vi "Main.vi"() -> ()   [LabVIEW 2018]
uses:
  MainFrame/TypeDefs/DisplayCluster.ctl
  MainFrame/TypeDefs/CiscoStats.ctl
  MainFrame/TypeDefs/Command_Enum.ctl
  ModulesDS/TypeDefs/PR_Parameters.ctl
  MainFrame/TypeDefs/FGV_Enum.ctl
  MainFrame/TypeDefs/InternalDataCluster.ctl
  Modules/Private Controls/Report Data Cluster.ctl
  Modules/Private Controls/Data Raw.ctl
  ModulesDS/GetNeglectedSRs.vi
  ModulesDS/GetOpenSRs.vi
  MainFrame/MainFrameLib.lvlib
  Modules/Data Operations.lvlib
  ModulesDS/SRReportParser.lvlib
  ModulesDS/SRNotesParser/SRNotesParser.lvlib
panel:
  in  "Tab Control":T1(tab)=enum."Debug\\Configure"
  in  "Stop":bool
  in  "Refresh CISCO Agents":bool
  out "AEs List":i32(listbox)
  in  "UpdateReports":bool
  in  "New AEs":string(combo)
  in  "Configure AE Name Mapping":bool
  in  "Cancel Request":bool
  in  "Clear Folder":bool
  out "Report Available":bool
  in  "Load existing report":bool
  in  "Request Oracle Report":bool
  out "Available weeks":string
  out "Request ID":string="45252303"
  out "Cisco Stats":T2[](array[typedef])=[{"Agent Name"="Akos Hegedus", "Number"="4091404", "State"="Logged Off", "Time in state"="-", "Ready ?"=FALSE}, {"Agent Name"="Alin Balanescu", "Number"="4091454", "State"="Ready", "Time in state"="01:06:36", "Ready ?"=TRUE}, {"Agent Name"="Ambrus Gregor", "Number"="4091431", "State"="Logged Off", "Time in state"="-", "Ready ?"=FALSE}, {"Agent Name"="Andrzej Filipek", "Number"="4091443", "State"="Ready", "Time in state"="00:16:58", "Ready ?"=TRUE}, {"Agent Name"="Denis Stavila", "Number"="4283512", "State"="Logged Off", "Time in state"="-", "Ready ?"=FALSE}, {"Agent Name"="Filip Pribyl", "Number"="4025617", "State"="Ready", "Time in state"="00:00:22", "Ready ?"=TRUE}, {"Agent Name"="Kamil Gierczyk", "Number"="4091512", "State"="Ready", "Time in state"="00:00:18", "Ready ?"=TRUE}, {"Agent Name"="Lukas Wiesner", "Number"="4023029", "State"="Logged Off", "Time in state"="-", "Ready ?"=FALSE}, {"Agent Name"="Michal Jadrny", "Number"="4025611", "State"="Logged Off", "Time in state"="-", "Ready ?"=FALSE}, {"Agent Name"="Patrik Karandusovsky", "Number"="4025621", "State"="Not Ready", "Time in state"="18:54:40", "Ready ?"=FALSE}, {"Agent Name"="Tamas Virag", "Number"="4091437", "State"="Ready", "Time in state"="00:07:00", "Ready ?"=TRUE}, {"Agent Name"="Tomasz Kachnic", "Number"="4091455", "State"="Logged Off", "Time in state"="-", "Ready ?"=FALSE}, {"Agent Name"="Tomasz Kowalczyk", "Number"="4091463", "State"="Ready", "Time in state"="00:17:46", "Ready ?"=TRUE}]
  out "Update Required?":bool
  out "State":T3=enum."Shutdown"
  in  "Available Reports":i32(listbox)=-1
  in  "Year":i16=1904 min=1904 max=1904 step=1
  in  "Week":i16 min=1 max=52 step=1
  in  "Excel Report":bool
  out "Open SRs":u32(colorbox)=16711680
  out "Solved in more then 5 workdays":u32(colorbox)=16753962
  out "In work":u32(colorbox)=9567230
  out "Solved within 5 workdays":u32(colorbox)=6618880
  out "New SRs":u32(colorbox)=16860
  out "SR Data":string[][](array[string])
  out "Data Display":T4[](array[typedef]) {"Open SRs" scale=0.0..40.0; "Solved in more then 5 Workdays" scale=0.0..40.0; "In Work SRs" scale=0.0..40.0; "Solved Within 5 workdays" scale=0.0..40.0; "New SRs" scale=0.0..40.0}
  in  "Team Stats":bool
  in  "SR Summary":string(tree)
  in  "Filter by AE Name":string(combo)="Alin Balanescu"
  in  "SaveNeglectedToFile":bool
  in  "Neglected SRs":string(tree)="3161536"
  in  "Open SRs":string(tree)="3191694"
  in  "AEs Overview":T5(array[cluster]) {"SRs # (Graphical)" max=350 step=1 scale=0.0..100.0}
  out "Documents Linked":string[][](table)
  out "Documents marked as solution":string[][](table)
  out "SR Notes":string[](array[string])
  in  "KCS Links":bool
  in  "SR View":string(tree)
  out "AE Statistics":string[][](table)
  in  "Get Performance Data":bool
  in  "Configuration":T6
  in  "EmailAddress:":string="tamas.virag@ni.com" caption="@ni.com"
  out "error out":errorcluster
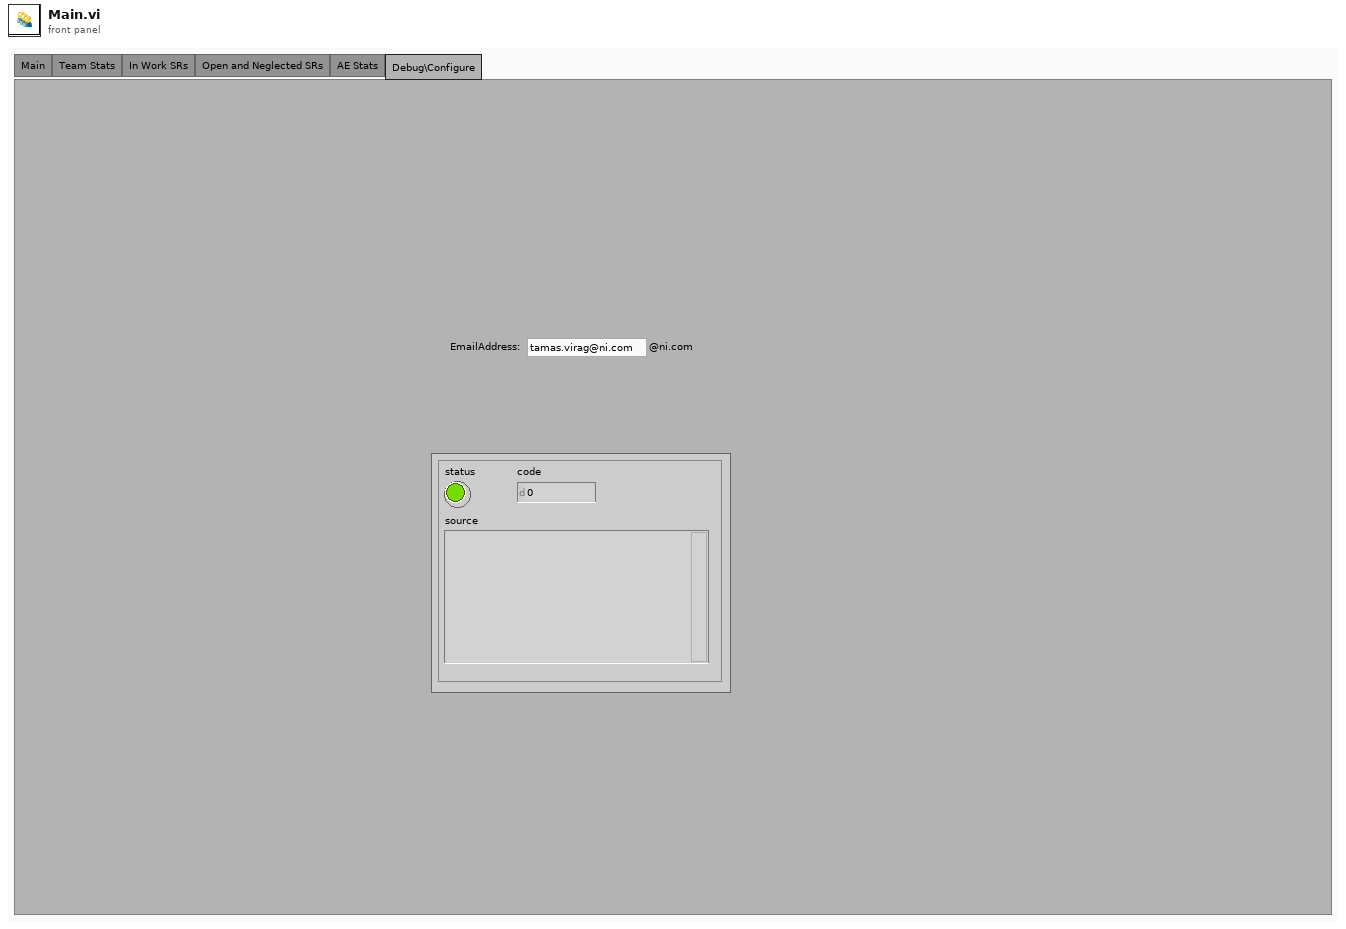
[diagram p1: front panel]
types:
  T1 = enum32{"Main", "Team Stats", "In Work SRs", "Open and Neglected SRs", "AE Stats", "Debug\\Configure"}
  T2 = typedef "MainFrameLib.lvlib/CiscoStats.ctl" = cluster{"Agent Name":string, "Number":string, "State":string, "Time in state":string, "Ready ?":bool}
  T3 = typedef "MainFrameLib.lvlib/Command_Enum.ctl" = enum16{"CheckSRLinks", "UpdateKCSColorCode", "StartLinkageCheck", "GetSRNotes", "DisplayAEStats", "InWork&Neglected", "RemapAENames", "ClearFolder", "UpdateReportsList", "ExcelReports", "TeamStats", "LoadReport", "WaitOnReport", "RequestReport", "Error", "Idle", "InitializeData", "ScreenPop", "Initialize", "UpdateCiscoAgentsView", "CancelRequests", "ClipboardCopy", "SaveNeglectedToFile", "Shutdown"}
  T4 = typedef "DS_Lib.lvlib/SRReportParser.lvlib/DisplayCluster.ctl" = cluster{"New SRs":u8, "Solved Within 5 workdays":u8, "In Work SRs":u8, "Solved in more then 5 Workdays":u8, "Open SRs":u8, "AE-Team":string}
  T5 = cluster{"AE Name":string, "SRs # (Graphical)":u16, "SRs #":dbl, "Solved within 5 business days #":string}[]
  T6 = typedef "DS_Lib.lvlib/SRReportParser.lvlib/PR_Parameters.ctl" = cluster{"AE":string, "Period":cluster{"Start Date":timestamp, "End Date":timestamp}}
  T7 = typedef "MainFrameLib.lvlib/InternalDataCluster.ctl" = cluster{"AE-Teams":string[], "AE-NamesMapping":cluster{"AE-Name(Raw)":string, "AE-Name (Proper)":string}[], "Report DVR":refnum<data-value>, "CISCO Agents":string[], "Controls":cluster{"Boolean":cluster{"Get Performance Data":refnum<vi>, "Request Oracle Report":refnum<vi>, "Refresh Button":refnum<vi>, "Load existing report":refnum<vi>, "Update Reports":refnum<vi>, "Configure AE Name Mapping":refnum<vi>, "Cancel Request":refnum<vi>, "KCS Links":refnum<vi>, "Team Stats":refnum<vi>, "Excel Report":refnum<vi>, "Clear Folder":refnum<vi>, "Report Available":refnum<vi>, "Update Required":refnum<vi>}, "Tree Controls":cluster{"Neglected SRs":refnum<vi>, "SR Summary":refnum<vi>, "Open SRs":refnum<vi>, "SR View":refnum<vi>}, "String Controls":cluster{"Available Weeks":refnum<vi>, "Request ID":refnum<vi>, "Filter AE by Name":refnum<vi>, "New AEs":refnum<vi>}, "Array Controls":cluster{"AEs Overview":refnum<vi>, "SR Data":refnum<vi>, "Data Display":refnum<vi>, "Cisco Stats":refnum<vi>}, "Table Controls":cluster{"AE Statistics":refnum<vi>}, "Color Boxes":cluster{"Open SRs":refnum<vi>, "Solved in more then 5 workdays":refnum<vi>, "Solved within 5 workdays":refnum<vi>, "in Work":refnum<vi>, "New SRs":refnum<vi>}, "Cluster Controls":cluster{"Configuration":refnum<vi>}, "Numeric Controls":cluster{"Available reports":refnum<vi>, "AEs List":refnum<vi>, "Year":refnum<vi>, "Week":refnum<vi>}, "Tab Control":cluster{"Tab Control":refnum<vi>}, "EmailAddress":refnum<vi>}}
  T8 = typedef "MainFrameLib.lvlib/FGV_Enum.ctl" = enum16{"Close", "GetRefs", "Initialize"}
  T9 = enum8{"Enabled", "Disabled", "Disabled and Grayed Out"}
  T10 = cluster{"Neglected SRs":refnum<vi>, "SR Summary":refnum<vi>, "Open SRs":refnum<vi>, "SR View":refnum<vi>}
  T11 = cluster{"AE-Name Raw":string, "AE-Name Proper":string}[]
  T12 = cluster{"AE-Name(Raw)":string, "AE-Name (Proper)":string}[]
  T13 = typedef "DS_Lib.lvlib/SRReportParser.lvlib/InWorkSR_Data.ctl" = cluster{"SR Number":string, "AE Owner":string, "Contact":string, "Summary":string, "Days since last update":dbl, "Status":string, "Neglected?":bool, "More then 5 business days ?":bool, "SurveyData":cluster{"Resolution Time":dbl, "Total Satisfaction":dbl, "Response Time":dbl, "Courtesy":dbl, "Problem Solved":dbl, "Level of effort":dbl}}
  T14 = cluster{"Start Date":timestamp, "End Date":timestamp}
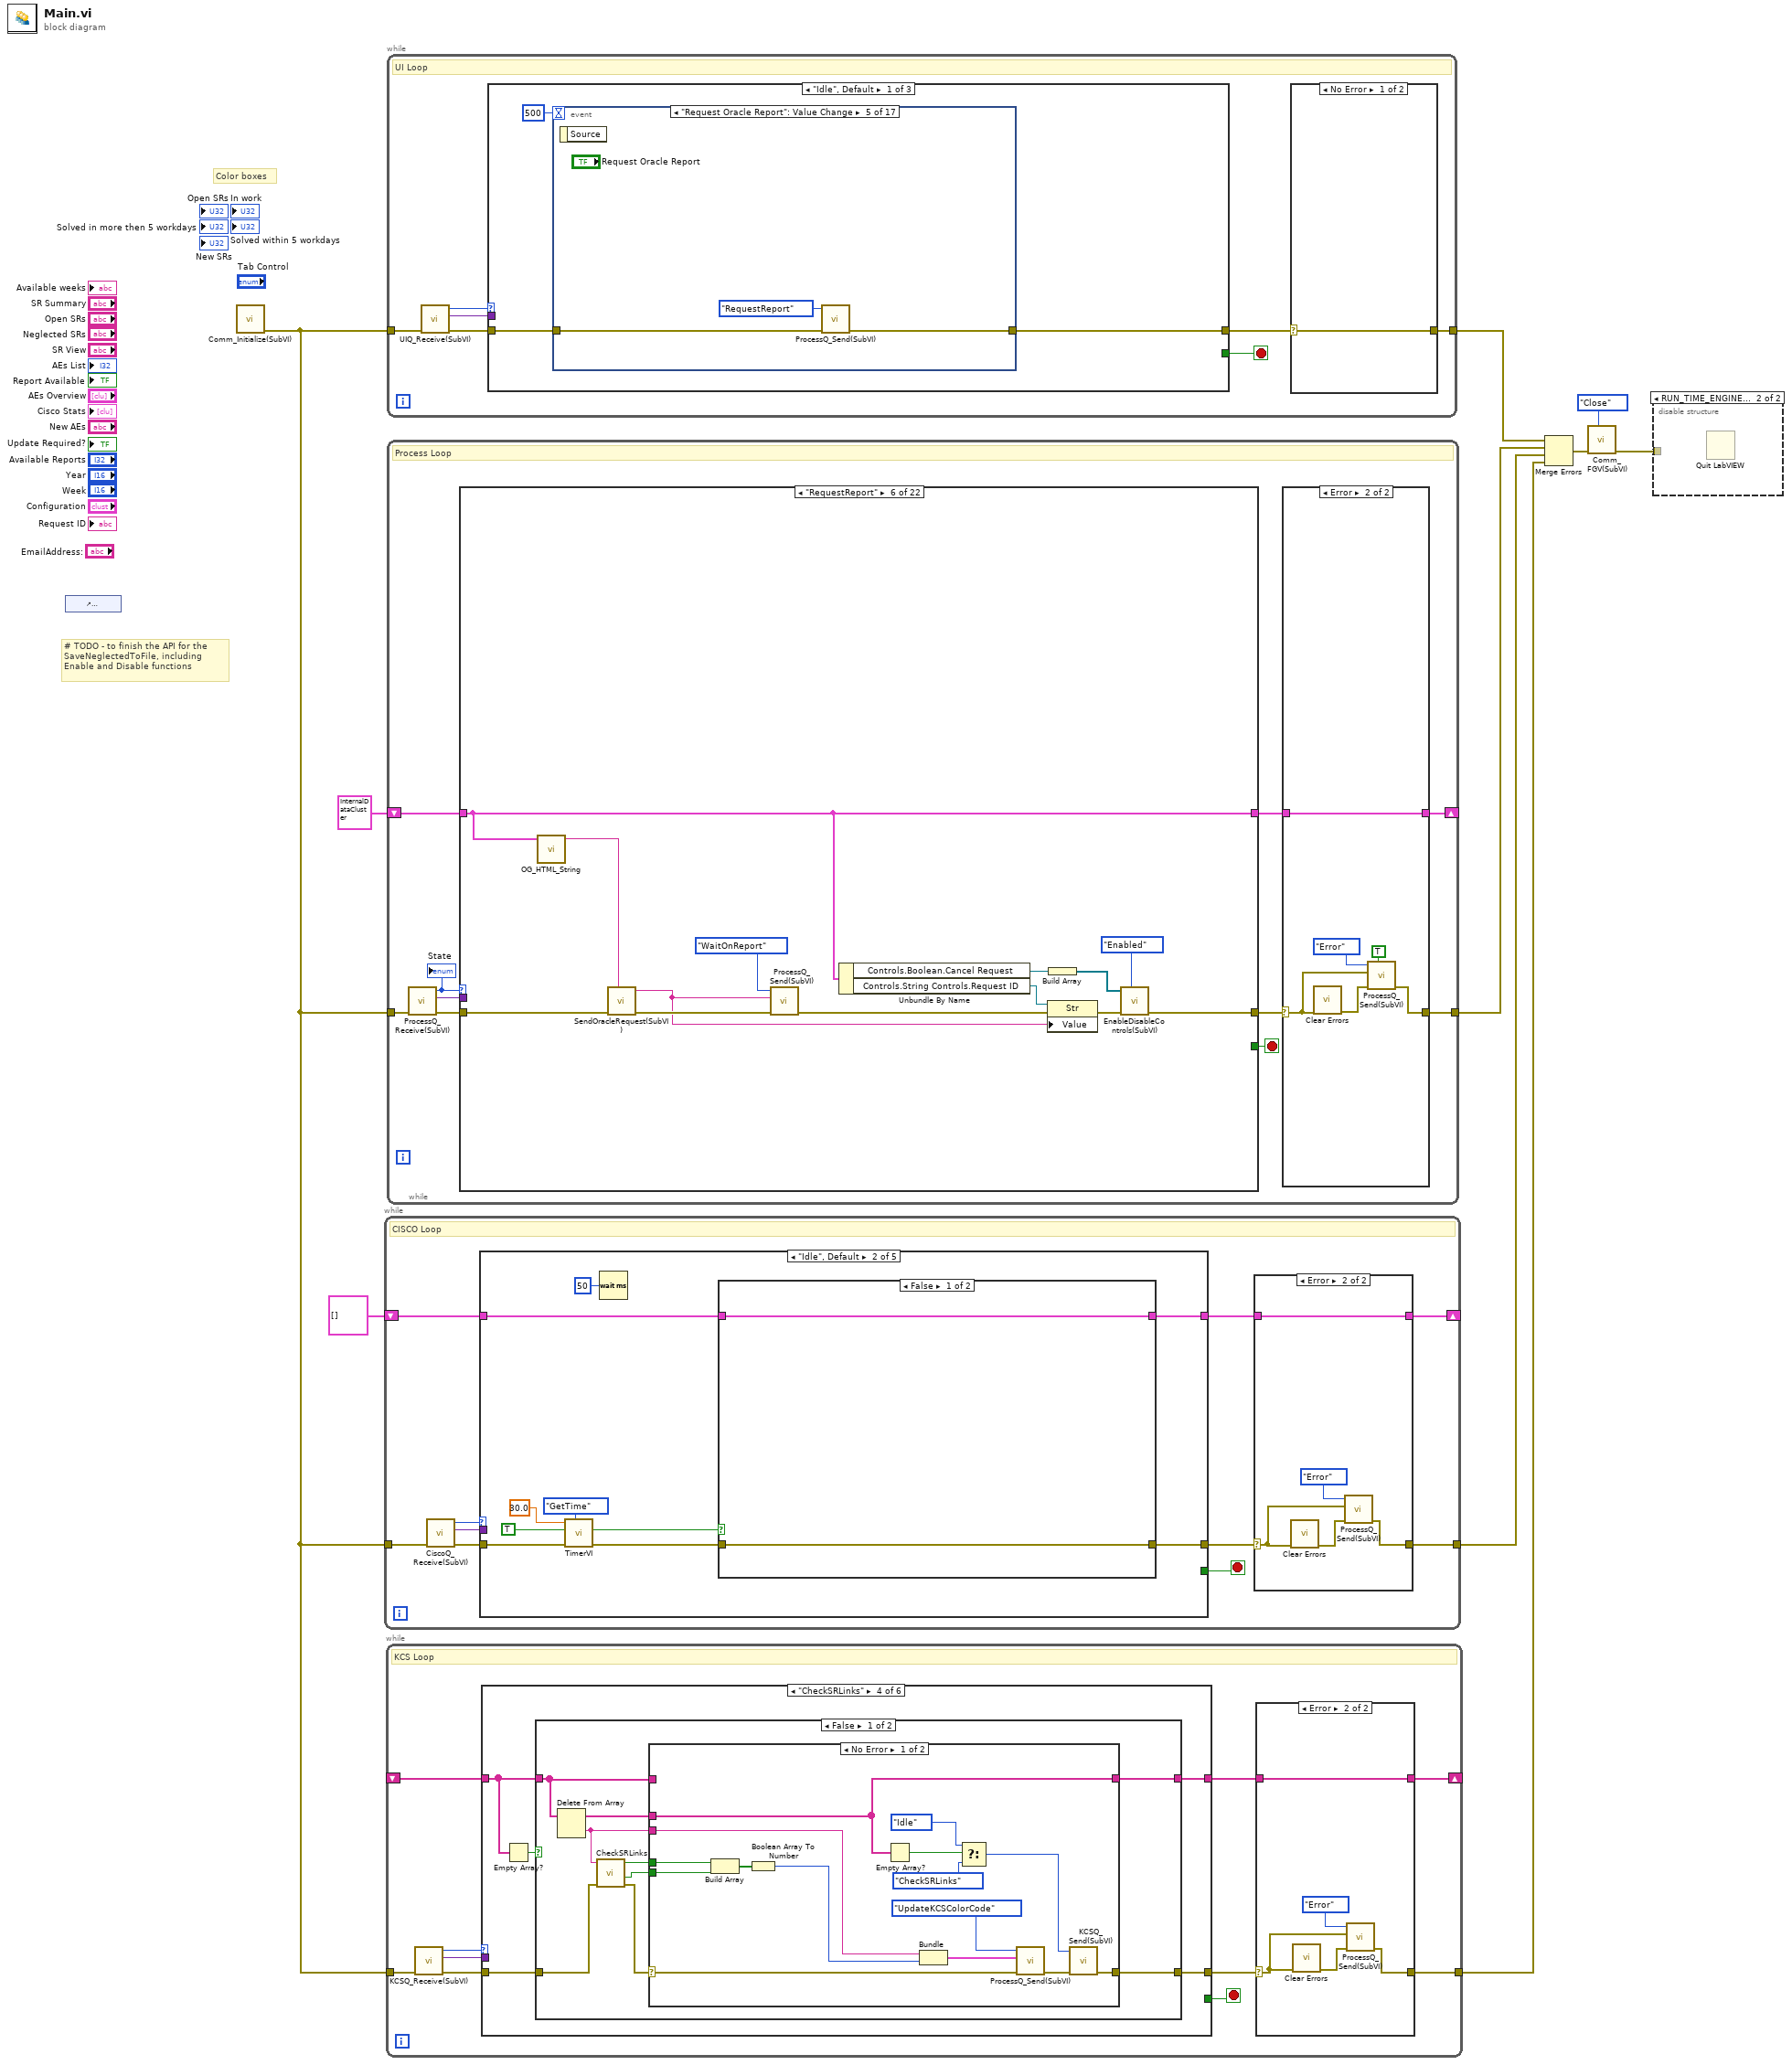
[diagram p0: block diagram]
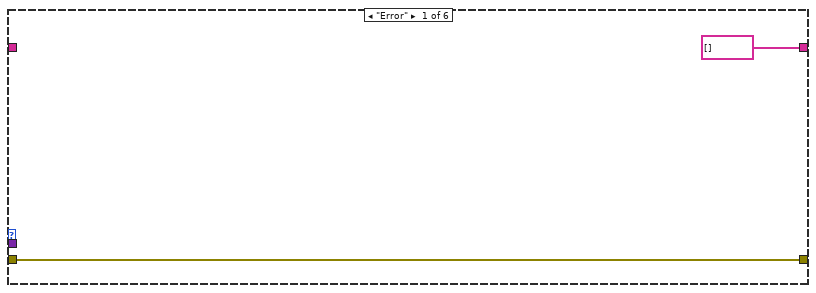
[diagram p3: hidden frame]
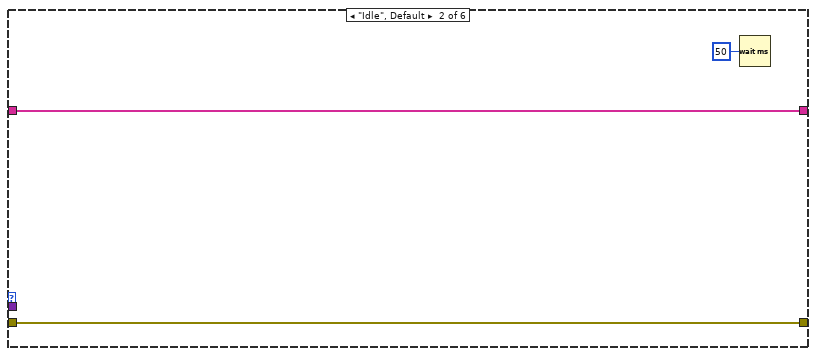
[diagram p4: hidden frame]
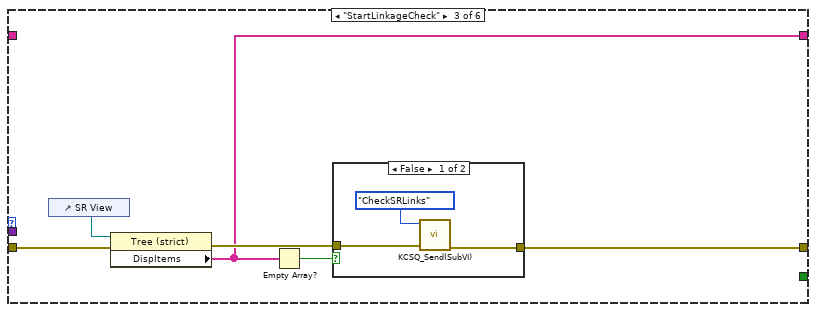
[diagram p5: hidden frame]
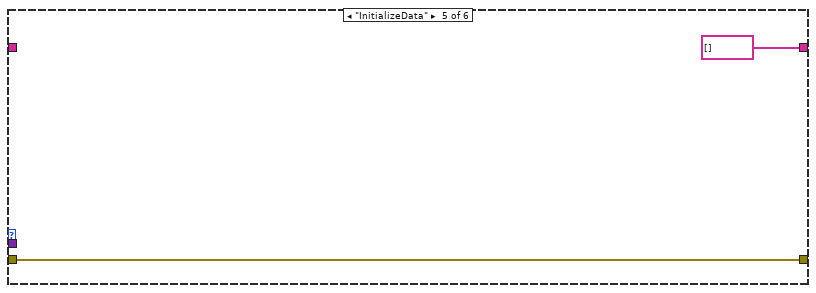
[diagram p9: hidden frame]
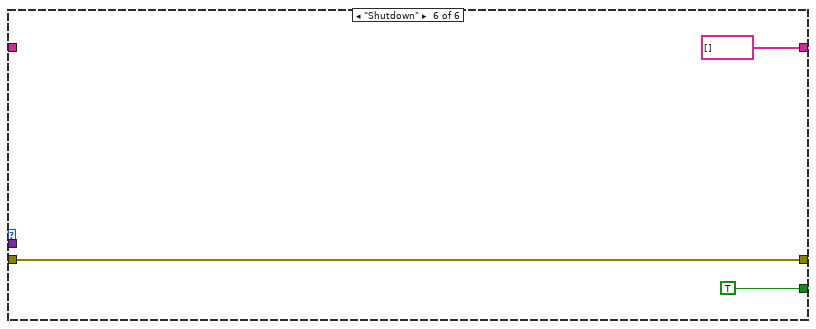
[diagram p10: hidden frame]
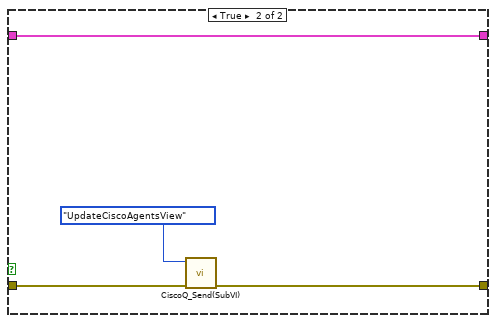
[diagram p14: hidden frame]
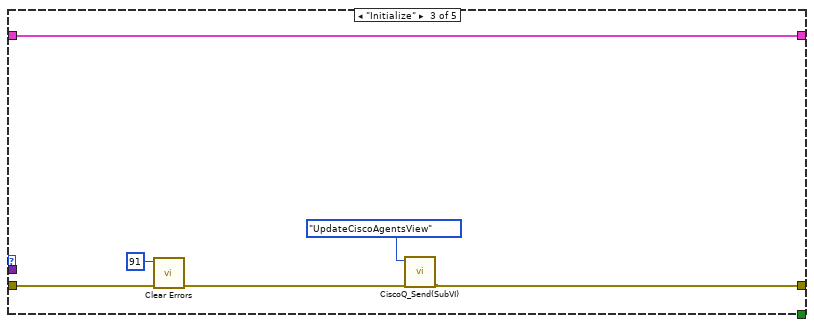
[diagram p15: hidden frame]
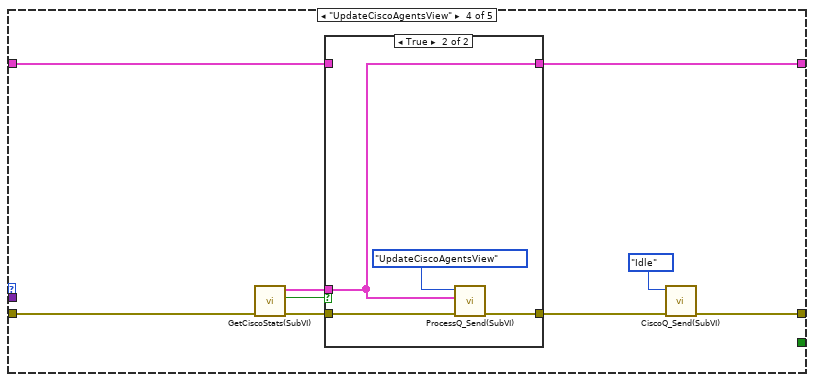
[diagram p16: hidden frame]
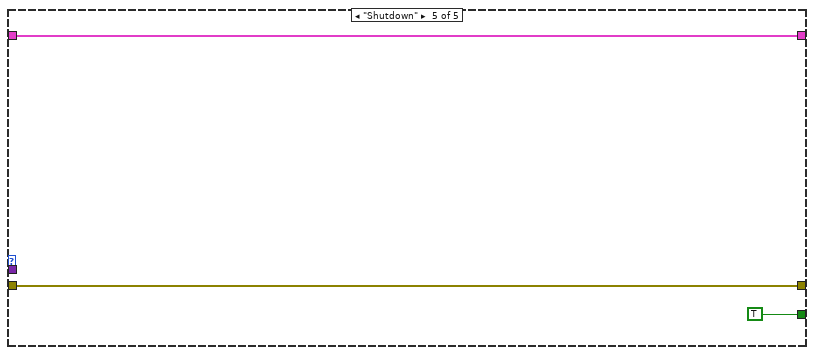
[diagram p18: hidden frame]
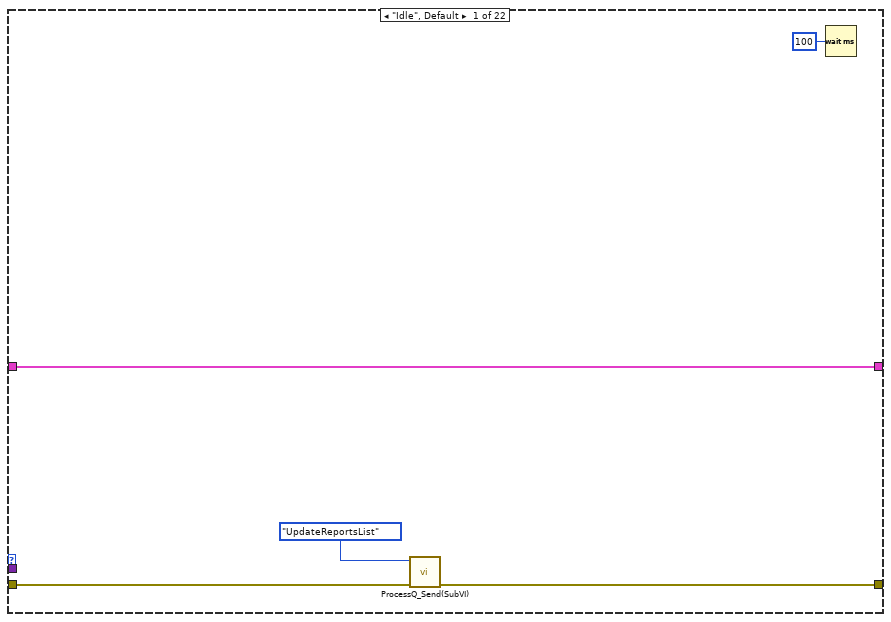
[diagram p20: hidden frame]
diagram:
  # "# TODO - to finish the API for the \nSaveNeglectedToFile, including \nEnable and Disable functions"
  # "Color boxes"
  n1 = control-ref of="SaveNeglectedToFile"() -> ()  [unwired: 1 out]
  n2 = call "Comm_Initialize(SubVI).vi"() -> ("error out"=w5:errorcluster)  [unwired: 11 in]
  n3 = while {
    tunnel: w5 -> [w20]
    tunnel: [w15] -> w4
    shift-right: [w11] -> _
    shift-left: T2[] [] ("Cisco Stats") -> [w14]
    stop <- w17 stop-if-true
    # "CISCO Loop"
    n4 = call "CiscoQ_Receive(SubVI).vi"("error in (no error)"=w20) -> ("error out"=w18:errorcluster, "Data"=w13:variant, "Command"=w19:T3)  [unwired: 8 in]
    n5 = case shown="\"Idle\", Default" w19 {
      tunnel: w18 -> [w29 w37 w46 w57 w67]
      tunnel: [w29 w39 w49 w53 w67] -> w16
      tunnel: [_ _ _ _ TRUE] -> w17
      tunnel: w14 -> [w28 w38 w47 w55 w68]
      tunnel: w13 -> [_ _ _ _ _]
      tunnel: [w28 w32 w47 w56 w68] -> w12
      frame "Error" {
      }
      frame "Idle", Default {
        n6 = call "TimerVI.vi"("Command"=enum16{"GetTime", "Reset"}."GetTime", "error in (no error)"=w37, "Autoreset ?"=TRUE ("Reset"), "Time Target (s)"=30.0) -> ("error out"=w36:errorcluster, "Time has elapsed?"=w31:bool)  [unwired: 5 in, 1 out]
        n7 = Wait (ms)(milliseconds to wait=u32 50) -> ()  [unwired: 1 out]
        n8 = case shown="False" w31 {
          tunnel: [w41 w43] -> w39
          tunnel: w36 -> [w41 w44]
          tunnel: w38 -> [w40 w45]
          tunnel: [w40 w45] -> w32
          frame False {
          }
          frame True {
            n9 = call "CiscoQ_Send(SubVI).vi"("error in (no error)"=w44, "Command"=Command_Enum."UpdateCiscoAgentsView") -> ("error out"=w43:errorcluster)  [unwired: 9 in]
          }
        }
      }
      frame "Initialize" {
        n10 = call <vilib>:"Clear Errors.vi"("error in (no error)"=w46, "specific error code to clear (0: all)"=91) -> ("error out"=w50:errorcluster)  [unwired: 4 in, 1 out]
        n11 = call "CiscoQ_Send(SubVI).vi"("error in (no error)"=w50, "Command"=Command_Enum."UpdateCiscoAgentsView") -> ("error out"=w49:errorcluster)  [unwired: 9 in]
      }
      frame "UpdateCiscoAgentsView" {
        n12 = call "GetCiscoStats(SubVI).vi"("error in (no error)"=w57) -> ("error IO"=w60:errorcluster, "Valid Data ?"=w59:bool, "Cisco Stats"=w58:T2[])  [unwired: 8 in]
        n13 = case shown="True" w59 {
          tunnel: w58 -> [_ w64]
          tunnel: w60 -> [w62 w66]
          tunnel: [w62 w65] -> w54
          tunnel: [w61 w64] -> w56
          tunnel: w55 -> [w61 _]
          frame False {
          }
          frame True {
            n14 = call "ProcessQ_Send(SubVI).vi"("error in (no error)"=w66, "Data"=w64, "Command"=Command_Enum."UpdateCiscoAgentsView") -> ("error out"=w65:errorcluster)  [unwired: 8 in]
          }
        }
        n15 = call "CiscoQ_Send(SubVI).vi"("error in (no error)"=w54, "Command"=Command_Enum."Idle") -> ("error out"=w53:errorcluster)  [unwired: 9 in]
      }
      frame "Shutdown" {
      }
    }
    n16 = case shown="Error" w16 {
      selector: w16 -> [w22 w24]
      tunnel: [w22 w25] -> w15
      tunnel: w12 -> [w21 w23]
      tunnel: [w21 w23] -> w11
      frame No Error {
      }
      frame Error {
        n17 = call <vilib>:"Clear Errors.vi"("error in (no error)"=w24) -> ("error out"=w26:errorcluster)  [unwired: 5 in, 1 out]
        n18 = call "ProcessQ_Send(SubVI).vi"("error in (no error)"=w26, "Data"=w24, "Command"=Command_Enum."Error") -> ("error out"=w25:errorcluster)  [unwired: 8 in]
      }
    }
  }
  n19 = while {
    tunnel: [w77] -> w3
    tunnel: w5 -> [w73]
    shift-right: [w71] -> _
    shift-left: _ -> [w70]
    stop <- w79 stop-if-true
    # "KCS Loop"
    n20 = call "KCSQ_Receive(SubVI).vi"("error in (no error)"=w73) -> ("error out"=w76:errorcluster, "Data"=w75:variant, "Command"=w74:T3)  [unwired: 8 in]
    n21 = case shown="\"CheckSRLinks\"" w74 {
      tunnel: w76 -> [w88 w91 w94 w106 w136 w139]
      tunnel: [w88 w91 w96 w102 w136 w139] -> w78
      tunnel: [_ _ _ _ _ TRUE] -> w79
      tunnel: w75 -> [_ _ _ _ _ _]
      tunnel: [string[] [] w90 w92 w103 string[] [] string[] []] -> w72
      tunnel: w70 -> [_ w90 _ w104 _ _]
      frame "Error" {
      }
      frame "Idle", Default {
        n22 = Wait (ms)(milliseconds to wait=u32 50) -> ()  [unwired: 1 out]
      }
      frame "StartLinkageCheck" {
        n23 = control-ref of="SR View"() -> (w95:refnum<vi>)
        n24 = property class="Tree (strict)"(reference=w95, error in=w94) -> (error out=w93:errorcluster, "DispItems"=w92:string[])  [unwired: 1 out]
        n25 = Empty Array?(array=w92) -> (empty?=w97:bool)
        n26 = case shown="False" w97 {
          tunnel: [w100 w101] -> w96
          tunnel: w93 -> [w98 w101]
          frame False {
            n27 = call "KCSQ_Send(SubVI).vi"("error in (no error)"=w98, "Command"=Command_Enum."CheckSRLinks") -> ("error out"=w100:errorcluster)  [unwired: 9 in]
          }
          frame True {
          }
        }
      }
      frame "CheckSRLinks" {
        n28 = Empty Array?(array=w104) -> (empty?=w105:bool)
        n29 = case shown="False" w105 {
          tunnel: w106 -> [w112 w134]
          tunnel: w104 -> [w115 w133]
          tunnel: [w108 w133] -> w103
          tunnel: [w107 w134] -> w102
          frame False {
            n30 = Delete From Array(array=w115) -> (deleted portion=w113:string, array with subset deleted=w114:string[])  [unwired: 2 in]
            n31 = call "CheckSRLinks.vi"("Error In"=w112, "SR #"=w113) -> ("Error Out"=w111:errorcluster, "Documents Used (B)"=w109:bool, "Documents Marked as Solution (B)"=w110:bool)  [unwired: 7 in]
            n32 = case shown="No Error" w111 {
              selector: w111 -> [w119 w131]
              tunnel: w115 -> [_ w132]
              tunnel: w114 -> [w126 _]
              tunnel: [w126 w132] -> w108
              tunnel: [w127 w131] -> w107
              tunnel: w113 -> [w121 _]
              tunnel: w110 -> [w129 _]
              tunnel: w109 -> [w128 _]
              frame No Error {
                n33 = Build Array(w129, w128) -> (w130:bool[])
                n34 = Boolean Array To Number(Boolean array=w130) -> (number=w120:u32)
                n35 = Empty Array?(array=w126) -> (empty?=w125:bool)
                n36 = Bundle(w121, w120) -> (w117:cluster{string, u32})  [unwired: 1 in]
                n37 = Select(t=Command_Enum."Idle" ("Command"), s=w125, f=Command_Enum."CheckSRLinks" ("Command")) -> (s? t:f=w122:T3)
                n38 = call "ProcessQ_Send(SubVI).vi"("error in (no error)"=w119, "Data"=w117, "Command"=Command_Enum."UpdateKCSColorCode") -> ("error out"=w118:errorcluster)  [unwired: 8 in]
                n39 = call "KCSQ_Send(SubVI).vi"("error in (no error)"=w118, "Command"=w122) -> ("error out"=w127:errorcluster)  [unwired: 9 in]
              }
              frame Error {
              }
            }
          }
          frame True {
          }
        }
      }
      frame "InitializeData" {
      }
      frame "Shutdown" {
      }
    }
    n40 = case shown="Error" w78 {
      selector: w78 -> [w81 w83]
      tunnel: [w81 w84] -> w77
      tunnel: w72 -> [w80 w82]
      tunnel: [w80 w82] -> w71
      frame No Error {
      }
      frame Error {
        n41 = call <vilib>:"Clear Errors.vi"("error in (no error)"=w83) -> ("error out"=w85:errorcluster)  [unwired: 5 in, 1 out]
        n42 = call "ProcessQ_Send(SubVI).vi"("error in (no error)"=w85, "Data"=w83, "Command"=Command_Enum."Error") -> ("error out"=w84:errorcluster)  [unwired: 8 in]
      }
    }
  }
  n43 = while {
    tunnel: [w146] -> w9
    tunnel: w5 -> [w144]
    stop <- w140 stop-if-true
    # "UI Loop"
    n44 = call "UIQ_Receive(SubVI).vi"("error in (no error)"=w144) -> ("error out"=w143:errorcluster, "Data"=w142:variant, "Command"=w145:T3)  [unwired: 8 in]
    n45 = case shown="\"Idle\", Default" w145 {
      tunnel: w143 -> [w148 w218 w221]
      tunnel: w142 -> [_ _ _]
      tunnel: [w147 w218 w220] -> w141
      tunnel: [_ _ TRUE] -> w140
      frame "Idle", Default {
        n46 = event shown="[4] \"Request Oracle Report\": Value Change" {
          selector: _ -> [_ _ _ _ _ _ _ _ _ _ _ _ _ _ _ _ _]
          dyn-events: _ -> [_ _ _ _ _ _ _ _ _ _ _ _ _ _ _ _ _]
          timeout: 500 -> [_ _ _ _ _ _ _ _ _ _ _ _ _ _ _ _ _]
          tunnel: [w150 w152 w154 w156 w158 w161 w164 w168 w171 w173 w179 w201 w203 w206 w209 w213 w216] -> w147
          tunnel: w148 -> [w150 w153 w155 w157 w159 w163 w165 w169 w172 w174 w177 w199 w204 w207 w210 w214 w217]
          event Timeout {
            n47 = event-data() -> ()  [unwired: 1 in, 3 out]
          }
          event "Refresh CISCO Agents": Value Change {
            n48 = event-data() -> ()  [unwired: 1 in, 1 out]
            n49 = call "CiscoQ_Send(SubVI).vi"("error in (no error)"=w153, "Command"=Command_Enum."UpdateCiscoAgentsView") -> ("error out"=w152:errorcluster)  [unwired: 9 in]
          }
          event Panel Close {
            n50 = event-data() -> ()  [unwired: 1 in, 1 out]
            n51 = call "Comm_Shutdown(SubVI).vi"("error in (no error)"=w155) -> ("error out"=w154:errorcluster)  [unwired: 10 in]
          }
          event "Stop": Value Change {
            n52 = event-data() -> ()  [unwired: 1 in, 6 out]
            n53 = call "Comm_Shutdown(SubVI).vi"("error in (no error)"=w157) -> ("error out"=w156:errorcluster)  [unwired: 10 in]
          }
          event "Request Oracle Report": Value Change {
            n54 = event-data() -> ()  [unwired: 1 in, 1 out]
            n55 = call "ProcessQ_Send(SubVI).vi"("error in (no error)"=w159, "Command"=Command_Enum."RequestReport") -> ("error out"=w158:errorcluster)  [unwired: 9 in]
          }
          event "Load existing report": Value Change {
            n56 = event-data() -> ()  [unwired: 1 in, 1 out]
            n57 = call "ProcessQ_Send(SubVI).vi"("error in (no error)"=w163, "Command"=Command_Enum."LoadReport") -> ("error out"=w161:errorcluster)  [unwired: 9 in]
          }
          event "UpdateReports": Value Change {
            n58 = event-data() -> ()  [unwired: 1 in, 6 out]
            n59 = call "ProcessQ_Send(SubVI).vi"("error in (no error)"=w165, "Command"=Command_Enum."UpdateReportsList") -> ("error out"=w164:errorcluster)  [unwired: 9 in]
          }
          event "Clear Folder": Value Change {
            n60 = event-data() -> ()  [unwired: 1 in, 1 out]
            n61 = call "ProcessQ_Send(SubVI).vi"("error in (no error)"=w169, "Command"=Command_Enum."ClearFolder") -> ("error out"=w168:errorcluster)  [unwired: 9 in]
          }
          event "Excel Report": Value Change {
            n62 = event-data() -> ()  [unwired: 1 in, 1 out]
            n63 = call "ProcessQ_Send(SubVI).vi"("error in (no error)"=w172, "Command"=Command_Enum."ExcelReports") -> ("error out"=w171:errorcluster)  [unwired: 9 in]
          }
          event "Team Stats": Value Change {
            n64 = event-data() -> ()  [unwired: 1 in, 6 out]
            n65 = call "ProcessQ_Send(SubVI).vi"("error in (no error)"=w174, "Command"=Command_Enum."TeamStats") -> ("error out"=w173:errorcluster)  [unwired: 9 in]
          }
          event "SR View", "Open SRs", "Neglected SRs", "SR Summary": Shortcut Menu Selection (User) {
            n66 = event-data() -> ("ItemTag"=w176:string, "CtlRef"=w178:refnum<vi>)  [unwired: 1 in]
            n67 = case shown="\"Copy SR#\"" w176 {
              tunnel: [w184 w186 w187 w197] -> w179
              tunnel: w178 -> [w183 _ w189 w196]
              tunnel: w177 -> [w182 w186 w188 w195]
              frame "Open ScreenPop" {
                n68 = property class="Tree (strict)"(reference=w183, error in=w182) -> (error out=w181:errorcluster, "Value"=w180:string)  [unwired: 1 out]
                n69 = call "ProcessQ_Send(SubVI).vi"("error in (no error)"=w181, "Data"=w180, "Command"=Command_Enum."ScreenPop") -> ("error out"=w184:errorcluster)  [unwired: 8 in]
              }
              frame "Something else", Default {
              }
              frame "SR Notes" {
                n70 = property class="Tree (strict)"(reference=w189, error in=w188) -> (error out=w191:errorcluster, "Value"=w190:string)  [unwired: 1 out]
                n71 = call "ProcessQ_Send(SubVI).vi"("error in (no error)"=w191, "Data"=w190, "Command"=Command_Enum."GetSRNotes") -> ("error out"=w187:errorcluster)  [unwired: 8 in]
              }
              frame "Copy SR#" {
                n72 = property class="Tree (strict)"(reference=w196, error in=w195) -> (error out=w194:errorcluster, "Value"=w193:string)  [unwired: 1 out]
                n73 = call "ProcessQ_Send(SubVI).vi"("error in (no error)"=w194, "Data"=w193, "Command"=Command_Enum."ClipboardCopy") -> ("error out"=w197:errorcluster)  [unwired: 8 in]
              }
            }
          }
          event "KCS Links": Value Change {
            n74 = event-data() -> ()  [unwired: 1 in, 1 out]
            n75 = call "KCSQ_Send(SubVI).vi"("error in (no error)"=w199, "Command"=Command_Enum."StartLinkageCheck") -> ("error out"=w201:errorcluster)  [unwired: 9 in]
          }
          event "Cancel Request": Value Change {
            n76 = event-data() -> ()  [unwired: 1 in, 6 out]
            n77 = call "ProcessQ_Send(SubVI).vi"("error in (no error)"=w204, "Command"=Command_Enum."CancelRequests") -> ("error out"=w203:errorcluster)  [unwired: 9 in]
          }
          event "Configure AE Name Mapping": Value Change {
            # "To be developed"
            n78 = event-data() -> ()  [unwired: 1 in, 6 out]
            n79 = call "ProcessQ_Send(SubVI).vi"("error in (no error)"=w207, "Command"=Command_Enum."RemapAENames") -> ("error out"=w206:errorcluster)  [unwired: 9 in]
          }
          event "Filter by AE Name": Value Change {
            n80 = event-data() -> ()  [unwired: 1 in, 6 out]
            n81 = call "ProcessQ_Send(SubVI).vi"("error in (no error)"=w210, "Data"="Filter by AE Name", "Command"=Command_Enum."InWork&Neglected") -> ("error out"=w209:errorcluster)  [unwired: 8 in]
          }
          event "SaveNeglectedToFile": Value Change {
            n82 = event-data() -> ()  [unwired: 1 in, 1 out]
            n83 = call "ProcessQ_Send(SubVI).vi"("error in (no error)"=w214, "Command"=Command_Enum."SaveNeglectedToFile") -> ("error out"=w213:errorcluster)  [unwired: 9 in]
          }
          event "Get Performance Data": Value Change {
            n84 = event-data() -> ()  [unwired: 1 in, 6 out]
            n85 = call "ProcessQ_Send(SubVI).vi"("error in (no error)"=w217, "Command"=Command_Enum."DisplayAEStats") -> ("error out"=w216:errorcluster)  [unwired: 9 in]
          }
        }
      }
      frame "InitializeData" {
      }
      frame "Shutdown" {
        n86 = call "ProcessQ_Send(SubVI).vi"("error in (no error)"=w221, "Command"=Command_Enum."Shutdown") -> ("error out"=w220:errorcluster)  [unwired: 9 in]
      }
    }
    n87 = case shown="No Error" w141 {
      selector: w141 -> [w223 w226]
      tunnel: [w223 w224] -> w146
      frame No Error {
      }
      frame Error {
        n88 = call <vilib>:"Clear Errors.vi"("error in (no error)"=w226) -> ("error out"=w225:errorcluster)  [unwired: 5 in, 1 out]
        n89 = call "ProcessQ_Send(SubVI).vi"("error in (no error)"=w225, "Data"=w226, "Command"=Command_Enum."Error") -> ("error out"=w224:errorcluster)  [unwired: 8 in]
      }
    }
  }
  n90 = while {
    tunnel: [w235] -> w10
    tunnel: w5 -> [w234]
    shift-right: [w229] -> _
    shift-left: T7 {"AE-Teams"=[], "AE-NamesMapping"=[], "Report DVR"=refnum, "CISCO Agents"=[], "Controls"={"Boolean"={"Get Performance Data"=refnum, "Request Oracle Report"=refnum, "Refresh Button"=refnum, "Load existing report"=refnum, "Update Reports"=refnum, "Configure AE Name Mapping"=refnum, "Cancel Request"=refnum, "KCS Links"=refnum, "Team Stats"=refnum, "Excel Report"=refnum, "Clear Folder"=refnum, "Report Available"=refnum, "Update Required"=refnum}, "Tree Controls"={"Neglected SRs"=refnum, "SR Summary"=refnum, "Open SRs"=refnum, "SR View"=refnum}, "String Controls"={"Available Weeks"=refnum, "Request ID"=refnum, "Filter AE by Name"=refnum, "New AEs"=refnum}, "Array Controls"={"AEs Overview"=refnum, "SR Data"=refnum, "Data Display"=refnum, "Cisco Stats"=refnum}, "Table Controls"={"AE Statistics"=refnum}, "Color Boxes"={"Open SRs"=refnum, "Solved in more then 5 workdays"=refnum, "Solved within 5 workdays"=refnum, "in Work"=refnum, "New SRs"=refnum}, "Cluster Controls"={"Configuration"=refnum}, "Numeric Controls"={"Available reports"=refnum, "AEs List"=refnum, "Year"=refnum, "Week"=refnum}, "Tab Control"={"Tab Control"=refnum}, "EmailAddress"=refnum}} -> [w231]
    stop <- w237 stop-if-true
    # "Process Loop"
    n91 = call "ProcessQ_Receive(SubVI).vi"("error in (no error)"=w234) -> ("error out"=w233:errorcluster, "Data"=w232:variant, "Command"=w228:T3)  [unwired: 8 in]
    "State" <- w228
    n92 = case shown="\"RequestReport\"" w228 {
      tunnel: [_ _ _ _ _ _ _ _ _ _ _ _ _ _ _ _ _ _ _ _ _ TRUE] -> w237
      tunnel: [w246 w251 w258 w270 w305 w357 w370 w451 w472 w483 w489 w496 w518 w533 w539 w555 w563 w578 w582 w592 w613 w640] -> w236
      tunnel: w233 -> [w247 w255 w259 w272 w327 w356 w372 w404 w463 w482 w494 w498 w515 w533 w542 w550 w568 w576 w585 w606 w620 w639]
      tunnel: w232 -> [_ w254 _ _ _ _ w371 w406 _ _ _ _ w531 _ _ _ w567 w573 w580 w605 w619 _]
      tunnel: w231 -> [w250 w253 w260 w274 w329 w351 w368 w427 w476 w481 w493 w505 w532 w534 w543 w562 w569 w579 w586 w601 w622 w642]
      tunnel: [w250 w253 w260 w273 w330 w351 w368 w448 w476 w481 w493 w505 w532 w534 w543 w562 w569 w579 w586 w604 w622 w642] -> w230
      frame "Idle", Default {
        n93 = call "ProcessQ_Send(SubVI).vi"("error in (no error)"=w247, "Command"=Command_Enum."UpdateReportsList") -> ("error out"=w246:errorcluster)  [unwired: 9 in]
        n94 = Wait (ms)(milliseconds to wait=u32 100) -> ()  [unwired: 1 out]
      }
      frame "Error" {
        n95 = Variant To Data(error in=w255, type=errorcluster {"status"=FALSE, "code"=0, "source"=""} ("error out"), Variant=w254) -> (data=→"error out":errorcluster, error out=w252:errorcluster)
        n96 = call "CommFlush(SubVI).vi"("error in (no error)"=w252) -> ("error out"=w251:errorcluster)  [unwired: 10 in]
      }
      frame "CancelRequests" {
        n97 = call "CommFlush(SubVI).vi"("error in (no error)"=w259) -> ("error out"=w258:errorcluster)  [unwired: 10 in]
      }
      frame "Initialize" {
        (unwired) T7 {"AE-Teams"=[], "AE-NamesMapping"=[], "Report DVR"=refnum, "CISCO Agents"=[], "Controls"={"Boolean"={"Get Performance Data"=refnum, "Request Oracle Report"=refnum, "Refresh Button"=refnum, "Load existing report"=refnum, "Update Reports"=refnum, "Configure AE Name Mapping"=refnum, "Cancel Request"=refnum, "KCS Links"=refnum, "Team Stats"=refnum, "Excel Report"=refnum, "Clear Folder"=refnum, "Report Available"=refnum, "Update Required"=refnum}, "Tree Controls"={"Neglected SRs"=refnum, "SR Summary"=refnum, "Open SRs"=refnum, "SR View"=refnum}, "String Controls"={"Available Weeks"=refnum, "Request ID"=refnum, "Filter AE by Name"=refnum, "New AEs"=refnum}, "Array Controls"={"AEs Overview"=refnum, "SR Data"=refnum, "Data Display"=refnum, "Cisco Stats"=refnum}, "Table Controls"={"AE Statistics"=refnum}, "Color Boxes"={"Open SRs"=refnum, "Solved in more then 5 workdays"=refnum, "Solved within 5 workdays"=refnum, "in Work"=refnum, "New SRs"=refnum}, "Cluster Controls"={"Configuration"=refnum}, "Numeric Controls"={"Available reports"=refnum, "AEs List"=refnum, "Year"=refnum, "Week"=refnum}, "Tab Control"={"Tab Control"=refnum}, "EmailAddress"=refnum}}
        n98 = control-ref of="Neglected SRs"() -> (w285:refnum<vi>)
        n99 = control-ref of="SR Summary"() -> (w286:refnum<vi>)
        n100 = control-ref of="Open SRs"() -> (w291:refnum<vi>)
        n101 = control-ref of="SR View"() -> (w287:refnum<vi>)
        n102 = control-ref of="Tab Control"() -> (w301:refnum<vi>)
        n103 = control-ref of="Filter by AE Name"() -> (w290:refnum<vi>)
        n104 = control-ref of="New AEs"() -> (w265:refnum<vi>)
        n105 = control-ref of="Open SRs"() -> (w294:refnum<vi>)
        n106 = control-ref of="Solved in more then 5 workdays"() -> (w295:refnum<vi>)
        n107 = control-ref of="New SRs"() -> (w296:refnum<vi>)
        n108 = control-ref of="Solved within 5 workdays"() -> (w297:refnum<vi>)
        n109 = control-ref of="In work"() -> (w298:refnum<vi>)
        n110 = control-ref of="Refresh CISCO Agents"() -> (w262:refnum<vi>)
        n111 = control-ref of="Update Required?"() -> (w267:refnum<vi>)
        n112 = control-ref of="Report Available"() -> (w268:refnum<vi>)
        n113 = control-ref of="Get Performance Data"() -> (w275:refnum<vi>)
        n114 = control-ref of="Request Oracle Report"() -> (w276:refnum<vi>)
        n115 = control-ref of="Load existing report"() -> (w277:refnum<vi>)
        n116 = control-ref of="UpdateReports"() -> (w278:refnum<vi>)
        n117 = control-ref of="Configure AE Name Mapping"() -> (w279:refnum<vi>)
        n118 = control-ref of="Cancel Request"() -> (w280:refnum<vi>)
        n119 = control-ref of="KCS Links"() -> (w281:refnum<vi>)
        n120 = control-ref of="Team Stats"() -> (w282:refnum<vi>)
        n121 = control-ref of="Excel Report"() -> (w283:refnum<vi>)
        n122 = control-ref of="Clear Folder"() -> (w284:refnum<vi>)
        n123 = control-ref of="Available Reports"() -> (w264:refnum<vi>)
        n124 = control-ref of="Configuration"() -> (w299:refnum<vi>)
        n125 = control-ref of="AEs List"() -> (w271:refnum<vi>)
        n126 = control-ref of="Cisco Stats"() -> (w266:refnum<vi>)
        n127 = control-ref of="Year"() -> (w263:refnum<vi>)
        n128 = control-ref of="Week"() -> (w300:refnum<vi>)
        n129 = control-ref of="Available weeks"() -> (w288:refnum<vi>)
        n130 = control-ref of="Request ID"() -> (w289:refnum<vi>)
        n131 = control-ref of="AEs Overview"() -> (w292:refnum<vi>)
        n132 = control-ref of="SR Data"() -> (w302:refnum<vi>)
        n133 = control-ref of="Data Display"() -> (w303:refnum<vi>)
        n134 = control-ref of="AE Statistics"() -> (w293:refnum<vi>)
        n135 = control-ref of="EmailAddress:"() -> (w261:refnum<vi>)
        n136 = Bundle By Name(cluster=w274, "Controls.Boolean.Update Required"=w267, "Controls.Boolean.Report Available"=w268, "Controls.Boolean.Get Performance Data"=w275, "Controls.Boolean.Request Oracle Report"=w276, "Controls.Boolean.Refresh Button"=w262, "Controls.Boolean.Load existing report"=w277, "Controls.Boolean.Update Reports"=w278, "Controls.Boolean.Configure AE Name Mapping"=w279, "Controls.Boolean.Cancel Request"=w280, "Controls.Boolean.KCS Links"=w281, "Controls.Boolean.Team Stats"=w282, "Controls.Boolean.Excel Report"=w283, "Controls.Boolean.Clear Folder"=w284, "Controls.Tree Controls.Neglected SRs"=w285, "Controls.Tree Controls.SR Summary"=w286, "Controls.Tree Controls.Open SRs"=w291, "Controls.Tree Controls.SR View"=w287, "Controls.String Controls.Available Weeks"=w288, "Controls.String Controls.Request ID"=w289, "Controls.String Controls.Filter AE by Name"=w290, "Controls.Array Controls.AEs Overview"=w292, "Controls.Array Controls.SR Data"=w302, "Controls.Array Controls.Data Display"=w303, "Controls.Table Controls.AE Statistics"=w293, "Controls.Color Boxes.Open SRs"=w294, "Controls.Color Boxes.Solved in more then 5 workdays"=w295, "Controls.Color Boxes.Solved within 5 workdays"=w296, "Controls.Color Boxes.in Work"=w297, "Controls.Color Boxes.New SRs"=w298, "Controls.Cluster Controls.Configuration"=w299, "Controls.Numeric Controls.Week"=w300, "Controls.Tab Control.Tab Control"=w301, "Controls.Numeric Controls.Available reports"=w264, "Controls.Numeric Controls.AEs List"=w271, "Controls.Array Controls.Cisco Stats"=w266, "Controls.String Controls.New AEs"=w265, "Controls.Numeric Controls.Year"=w263, "Controls.EmailAddress"=w261) -> (w273:T7)
        n137 = call "ProcessQ_Send(SubVI).vi"("error in (no error)"=w272, "Command"=Command_Enum."InitializeData") -> ("error out"=w270:errorcluster)  [unwired: 9 in]
      }
      frame "InitializeData" {
        # "# TODO Check the CmbBox Error\nAdded a ClearErrors VI to temporarily get rid of it"
        n138 = Unbundle By Name(w329) -> ("Controls.Numeric Controls.Available reports"=w311:refnum<vi>, "Controls.Numeric Controls.AEs List"=w334:refnum<vi>, "Controls.Cluster Controls.Configuration"=w336:refnum<vi>, "Controls.String Controls.Filter AE by Name"=w337:refnum<vi>)
        n139 = Unbundle By Name(w329) -> ("Controls.Boolean.Get Performance Data"=w346:refnum<vi>, "Controls.Boolean.Configure AE Name Mapping"=w345:refnum<vi>, "Controls.Boolean.Cancel Request"=w344:refnum<vi>, "Controls.Boolean.KCS Links"=w343:refnum<vi>, "Controls.Boolean.Team Stats"=w342:refnum<vi>, "Controls.Boolean.Excel Report"=w341:refnum<vi>)
        n140 = Unbundle By Name(w329) -> ("Controls.Boolean.Report Available"=w315:refnum<vi>, "Controls.Numeric Controls.Available reports"=w328:refnum<vi>)
        n141 = call "GetReportsList(SubVI).vi"("error in (no error)"=w327) -> ("error out"=w325:errorcluster, "Available Reports"=w338:string[])  [unwired: 9 in]
        n142 = Unbundle By Name(w329) -> ("Controls.Tree Controls"=w349:T10)
        n143 = Cluster To Array(cluster=w349) -> (array=w348:refnum<vi>[])
        n144 = call "NameMapping_read.vi"("error in (no error)"=w327) -> ("error out"=w326:errorcluster, "AE-Names Mapping"=w332:T11, "AE-Names (Filter)"=w333:cluster{"String":string, "String":string}[], "AE-List"=w316:string[])  [unwired: 7 in]
        n145 = call "ClearTreeControls (SubVI).vi"("error in (no error)"=w327, "Tree Control Refnums"=w348) -> ("error out"=w347:errorcluster)  [unwired: 9 in]
        n146 = property class="LstBox (strict)"(reference=w328, error in=w325, "Item Names"=w338) -> (error out=w314:errorcluster)  [unwired: 1 out]
        n147 = Build Array(w346, w345, w344, w343, w342, w341) -> (w340:refnum<vi>[])
        n148 = call "GetConfigurationComboBox(SubVI).vi"("Cluster in"=w336) -> ("ComboBox out"=w335:refnum<vi>)  [unwired: 10 in]
        n149 = property class="LstBox (strict)"(reference=w311, "Value"=0) -> (error out=w309:errorcluster)  [unwired: 1 in, 1 out]
        n150 = property class="CmbBox"(reference=w337, error in=w326, "Strings And Values[]"=w333) -> (error out=w321:errorcluster)  [unwired: 1 out]
        n151 = property class="CmbBox"(reference=w335, error in=w326, "Strings And Values[]"=w333) -> (error out=w322:errorcluster)  [unwired: 1 out]
        n152 = property class="LstBox (strict)"(reference=w334, error in=w326, "Item Names"=w316) -> (error out=w323:errorcluster)  [unwired: 1 out]
        n153 = call "EnableDisableControls(SubVI).vi"("Enabled ?"=T9."Disabled and Grayed Out", "error in (no error)"=w347, "References Array"=w340) -> ("error out"=w324:errorcluster)  [unwired: 8 in]
        n154 = property class="Bool (strict)"(reference=w315, error in=w314, "Value"=FALSE) -> (error out=w313:errorcluster)  [unwired: 1 out]
        n155 = Merge Errors(w309, w323, w322, w321) -> (w320:errorcluster)
        n156 = Merge Errors(w320, w324, w313) -> (w308:errorcluster)
        n157 = call <vilib>:"Clear Errors.vi"("error in (no error)"=w308) -> ("error out"=w307:errorcluster)  [unwired: 5 in, 1 out]
        n158 = call "NameMapping_read.vi"("error in (no error)"=w307) -> ("error out"=w317:errorcluster, "AE-List"=w318:string[])  [unwired: 7 in, 2 out]
        n159 = Bundle By Name(cluster=w329, "CISCO Agents"=w316, "AE-Teams"=string[] ["AE-Poland", "AE-Czech Republic and AE-Slovakia", "AE-Hungary", "AE-Romania"], "AE-NamesMapping"=w332) -> (w330:T7)
        n160 = call "CiscoQ_Send(SubVI).vi"("error in (no error)"=w317, "Data"=w318, "Command"=Command_Enum."Initialize") -> ("error out"=w306:errorcluster)  [unwired: 8 in]
        n161 = call "ProcessQ_Send(SubVI).vi"("error in (no error)"=w306, "Command"=Command_Enum."UpdateReportsList") -> ("error out"=w305:errorcluster)  [unwired: 9 in]
      }
      frame "RequestReport" {
        n162 = call "OG_HTML_String.vi"("Cluster"=w351) -> ("String"=w350:string)  [unwired: 10 in]
        n163 = call "SendOracleRequest(SubVI).vi"("HTTP string"=w350, "error in (no error)"=w356) -> ("error out"=w361:errorcluster, "Request ID"=w352:string)  [unwired: 8 in]
        n164 = call "ProcessQ_Send(SubVI).vi"("error in (no error)"=w361, "Data"=w352, "Command"=Command_Enum."WaitOnReport") -> ("error out"=w355:errorcluster)  [unwired: 8 in]
        n165 = Unbundle By Name(w351) -> ("Controls.Boolean.Cancel Request"=w360:refnum<vi>, "Controls.String Controls.Request ID"=w354:refnum<vi>)
        n166 = property class="Str"(reference=w354, error in=w355, "Value"=w352) -> (error out=w353:errorcluster)  [unwired: 1 out]
        n167 = Build Array(w360) -> (w359:refnum<vi>[])
        n168 = call "EnableDisableControls(SubVI).vi"("Enabled ?"=T9."Enabled", "error in (no error)"=w353, "References Array"=w359) -> ("error out"=w357:errorcluster)  [unwired: 8 in]
      }
      frame "WaitOnReport" {
        n169 = call <vilib>:"Application Directory.vi"() -> ("Application Directory"=w377:path)
        n170 = Variant To Data(error in=w372, type="", Variant=w371) -> (data=w365:string, error out=w375:errorcluster)
        n171 = Build Path(base path=w377, name or relative path="SurveyData") -> (appended path=w378:path)
        n172 = List Folder(path=w378, error in=w375) -> (filenames=w374:string[], error out=w364:errorcluster)  [unwired: 2 in, 2 out]
        n173 = for {
          tunnel: w374 -> [w400] mode=indexing
          tunnel: w365 -> [w399]
          tunnel: [w397] -> w373 mode=indexing
          n174 = Match Pattern(string=w400, regular expression=w399) -> (offset past match=w398:i32)  [unwired: 1 in, 3 out]
          n175 = Greater Or Equal To 0?(x=w398) -> (x >= 0?=w397:bool)
        }
        n176 = Unbundle By Name(w368) -> ("Controls.Boolean.Cancel Request"=w367:refnum<vi>, "Controls.Boolean.Report Available"=w363:refnum<vi>)
        n177 = Or Array Elements(Boolean array=w373) -> (logical OR=w369:bool)
        n178 = case shown="True" w369 {
          tunnel: [w382 w393] -> w370
          tunnel: w367 -> [_ w392]
          tunnel: w365 -> [w384 w391]
          tunnel: w364 -> [w385 w388]
          tunnel: w363 -> [w381 _]
          frame False {
            n179 = call "ProcessQ_Send(SubVI).vi"("error in (no error)"=w385, "Data"=w384, "Command"=Command_Enum."WaitOnReport") -> ("error out"=w383:errorcluster)  [unwired: 8 in]
            n180 = property class="Bool (strict)"(reference=w381, error in=w383, "Value"=FALSE) -> (error out=w382:errorcluster)  [unwired: 1 out]
          }
          frame True {
            n181 = call "ProcessQ_Send(SubVI).vi"("error in (no error)"=w388, "Command"=Command_Enum."UpdateReportsList") -> ("error out"=w387:errorcluster)  [unwired: 9 in]
            n182 = Build Array(w392) -> (w395:refnum<vi>[])
            n183 = call "ProcessQ_Send(SubVI).vi"("error in (no error)"=w387, "Data"=w391, "Command"=Command_Enum."LoadReport") -> ("error out"=w389:errorcluster)  [unwired: 8 in]
            n184 = call "EnableDisableControls(SubVI).vi"("Enabled ?"=T9."Disabled and Grayed Out", "error in (no error)"=w389, "References Array"=w395) -> ("error out"=w393:errorcluster)  [unwired: 8 in]
          }
        }
        n185 = Wait (ms)(milliseconds to wait=u32 50) -> ()  [unwired: 1 out]
      }
      frame "LoadReport" {
        w420 = "%Y" ("time format string (%c)")
        n186 = Unbundle By Name(w427) -> ("Controls.Numeric Controls.Year"=w425:refnum<vi>, "Controls.Numeric Controls.Week"=w416:refnum<vi>, "AE-NamesMapping"=w426:T12, "Controls.Numeric Controls.Available reports"=w435:refnum<vi>, "Report DVR"=w449:refnum<data-value>)
        n187 = Unbundle By Name(w427) -> ("Controls.Boolean.Report Available"=w439:refnum<vi>, "Controls.Boolean.Get Performance Data"=w447:refnum<vi>, "Controls.Boolean.Configure AE Name Mapping"=w446:refnum<vi>, "Controls.Boolean.KCS Links"=w445:refnum<vi>, "Controls.Boolean.Team Stats"=w444:refnum<vi>, "Controls.Boolean.Excel Report"=w443:refnum<vi>)
        n188 = Variant To Data(error in=w404, type="", Variant=w406) -> (data=w402:string, error out=w403:errorcluster)
        n189 = call "CloseSRDataReference(SubVI).vi"("error in (no error)"=w404, "Report DVR"=w449) -> ("error out"=w434:errorcluster)  [unwired: 9 in]
        n190 = case shown="Error" w403 {
          tunnel: [w457 w462] -> w436
          tunnel: w435 -> [_ w461]
          tunnel: w434 -> [w457 w460]
          tunnel: w402 -> [w458 _]
          tunnel: [w458 w459] -> w401
          frame No Error {
          }
          frame Error {
            n191 = call "GetReportSelection(SubVI).vi"("error in (no error)"=w460, "ListBox in"=w461) -> ("error out"=w462:errorcluster, "Selected Report"=w459:string)  [unwired: 8 in]
          }
        }
        n192 = call "FindReport (SubVI).vi"("error in (no error)"=w436, "ReportID"=w401) -> ("error out"=w452:errorcluster, "Report path"=w456:path)  [unwired: 8 in]
        n193 = call "ReadReport.vi"("error in (no error)"=w452, "FILE PATH TO REPORT DATA"=w456) -> ("error out"=w440:errorcluster, "DVR Out"=w455:refnum<data-value>)  [unwired: 8 in]
        n194 = call "FilterSRsStats(SubVI).vi"("Filter Parameters"=string[] ["Created in Error", "Declined to Purchase Support", "Expired", "Forum Resolved Customer", "RMA In Progress", "RMA Open", "Status"], "error in (no error)"=w440, "Data Value Reference in"=w455) -> ("error out"=w432:errorcluster, "Data Value Reference out"=w433:refnum<data-value>)  [unwired: 6 in, 1 out]
        n195 = call "UpdateAENames(SubVI).vi"("error in (no error)"=w432, "AE-NamesMapping"=w426, "Data Value Reference In"=w433) -> ("error out"=w430:errorcluster, "Data Value Reference out"=w431:refnum<data-value>)  [unwired: 7 in]
        n196 = Build Array(w447, w446, w445, w444, w443) -> (w442:refnum<vi>[])
        n197 = call "UpdateWeeks (SubVI).vi"("Error In"=w430, "DVR In"=w431) -> ("Error Out"=w428:errorcluster, "End Date"=w417:timestamp, "Start Date"=w423:timestamp, "DVR Out"=w429:refnum<data-value>)  [unwired: 6 in]
        n198 = Not(x=w428) -> (.not. x?=w438:bool)
        n199 = Format Date/Time String(time format string (%c)=w420, seconds (now)=w417) -> (date/time string=w421:string)  [unwired: 1 in]
        n200 = call "EnableDisableControls(SubVI).vi"("Enabled ?"=T9."Enabled", "error in (no error)"=w428, "References Array"=w442) -> ("error out"=w411:errorcluster)  [unwired: 8 in]
        n201 = Format Date/Time String(time format string (%c)=w420, seconds (now)=w423) -> (date/time string=w424:string)  [unwired: 1 in]
        n202 = Format Date/Time String(time format string (%c)="%W", seconds (now)=w417) -> (date/time string=w418:string)  [unwired: 1 in]
        n203 = property class="Bool (strict)"(reference=w439, error in=w428, "Value"=w438) -> (error out=w437:errorcluster)  [unwired: 1 out]
        n204 = Decimal String To Number(string=w421) -> (number=w419:i32)  [unwired: 2 in, 1 out]
        n205 = Decimal String To Number(string=w424) -> (number=w422:i32)  [unwired: 2 in, 1 out]
        n206 = Decimal String To Number(string=w418) -> (number=w415:i32)  [unwired: 2 in, 1 out]
        n207 = call "ProcessQ_Send(SubVI).vi"("error in (no error)"=w411, "Command"=Command_Enum."TeamStats") -> ("error out"=w410:errorcluster)  [unwired: 9 in]
        n208 = property class="DigNum (strict)"(reference=w425, "Minimum"=w422, "Maximum"=w419, "Value"=w419) -> (error out=w412:errorcluster)  [unwired: 1 in, 1 out]
        n209 = property class="DigNum (strict)"(reference=w416, "Value"=w415) -> (error out=w413:errorcluster)  [unwired: 1 in, 1 out]
        n210 = call "ProcessQ_Send(SubVI).vi"("error in (no error)"=w410, "Command"=Command_Enum."InWork&Neglected") -> ("error out"=w409:errorcluster)  [unwired: 9 in]
        n211 = Bundle By Name(cluster=w427, "Report DVR"=w429) -> (w448:T7)
        n212 = call "ProcessQ_Send(SubVI).vi"("error in (no error)"=w409, "Command"=Command_Enum."UpdateReportsList") -> ("error out"=w407:errorcluster)  [unwired: 9 in]
        n213 = Merge Errors(w412, w413, w437, w407) -> (w451:errorcluster)
      }
      frame "TeamStats" {
        n214 = Unbundle By Name(w476) -> ("Report DVR"=w471:refnum<data-value>, "AE-Teams"=w475:string[], "Controls.Numeric Controls.Week"=w470:refnum<vi>, "Controls.Numeric Controls.Year"=w468:refnum<vi>)
        n215 = property class="DigNum (strict)"(reference=w470, error in=w463) -> (error out=w466:errorcluster, "Value"=w469:i16)  [unwired: 1 out]
        n216 = property class="DigNum (strict)"(reference=w468, error in=w463) -> (error out=w465:errorcluster, "Value"=w467:i16)  [unwired: 1 out]
        n217 = Merge Errors(w466, w465) -> (w464:errorcluster)
        n218 = call "AE Groups SR Data.vi"("Year"=w467, "Week"=w469, "error in (no error)"=w464, "AE-Groups In"=w475, "Report DVR in"=w471) -> ("error out"=w472:errorcluster, "Formated SR Data Out"=→"SR Data":string[][], "SRs Out"=→"Data Display":T4[])  [unwired: 3 in, 1 out]
      }
      frame "ExcelReports" {
        n219 = Unbundle By Name(w481) -> ("Report DVR"=w485:refnum<data-value>, "AE-Teams"=w487:string[])
        n220 = Unbundle By Name(w481) -> ("Controls.Numeric Controls.Week"=w480:refnum<vi>, "Controls.Numeric Controls.Year"=w478:refnum<vi>)
        n221 = property class="DigNum (strict)"(reference=w478) -> ("Value"=w477:i16)  [unwired: 1 in, 2 out]
        n222 = property class="DigNum (strict)"(reference=w480) -> ("Value"=w479:i16)  [unwired: 1 in, 2 out]
        n223 = call "AE Groups SR Data.vi"("Year"=w477, "Week"=w479, "error in (no error)"=w482, "AE-Groups In"=w487, "Report DVR in"=w485) -> ("error out"=w484:errorcluster, "Formated SR Data Out"=w486:string[][])  [unwired: 3 in, 2 out]
        n224 = call "ToExcelTemplate.vi"("Repport Type"=enum16{"Weekly SR Data", "SR Trends"}."Weekly SR Data", "error in (no error)"=w484, "Data In"=w486) -> ("error out"=w483:errorcluster)  [unwired: 6 in, 2 out]
      }
      frame "UpdateReportsList" {
        n225 = call "GetReportsList(SubVI).vi"("error in (no error)"=w494) -> ("error out"=w492:errorcluster, "Available Reports"=w490:string[])  [unwired: 9 in]
        n226 = Unbundle By Name(w493) -> ("Controls.Numeric Controls.Available reports"=w491:refnum<vi>)
        n227 = property class="LstBox (strict)"(reference=w491, error in=w492, "Item Names"=w490) -> (error out=w489:errorcluster)  [unwired: 1 out]
      }
      frame "ClearFolder" {
        n228 = call <vilib>:"Application Directory.vi"() -> ("Application Directory"=w504:path)
        n229 = Build Path(base path=w504, name or relative path="SurveyData") -> (appended path=w503:path)
        n230 = List Folder(path=w503, error in=w498) -> (path out=w502:path, filenames=w500:string[], error out=w501:errorcluster)  [unwired: 2 in, 1 out]
        n231 = for {
          tunnel: w502 -> [w510]
          tunnel: w500 -> [w509] mode=indexing
          shift-right: [w506] -> w497
          shift-left: w501 -> [w507]
          n232 = Build Path(base path=w510, name or relative path=w509) -> (appended path=w508:path)
          n233 = Delete(path (use dialog)=w508, error in=w507) -> (error out=w506:errorcluster)  [unwired: 3 in, 2 out]
        }
        n234 = call "ProcessQ_Send(SubVI).vi"("error in (no error)"=w497, "Command"=Command_Enum."UpdateReportsList") -> ("error out"=w496:errorcluster)  [unwired: 9 in]
      }
      frame "InWork&Neglected" {
        w512 = ""
        n235 = Unbundle By Name(w532) -> ("Report DVR"=w516:refnum<data-value>)
        n236 = Variant To Data(error in=w515, type=w512, Variant=w531) -> (data=w513:string, error out=w514:errorcluster)
        n237 = Select(t=w512, s=w514, f=w513) -> (s? t:f=w511:string)
        n238 = call "GetSRsbyStatus.vi"("Statuses"=string[] ["IN WORK Escalation", "IN WORK", "RMA In Progress", "IN WORK Wait on Customer", "IN WORK Collab with PSE", "RMA Waiting on Customer", "RMA Open"], "Error In"=w515, "Report DVR in"=w516) -> ("Error Out"=w523:errorcluster, "SRs Out"=w524:T13[])  [unwired: 6 in, 1 out]
        n239 = call-poly "SelectsSRs(Poly).vi"("error in (no error)"=w523, "SRs Array"=w524) -> ("error out"=w526:errorcluster, "Open SRs"=w525:T13[])  [unwired: 6 in]
        n240 = call-poly "SelectsSRs(Poly).vi"("error in (no error)"=w523, "SRs Array"=w524) -> ("error out"=w522:errorcluster, "Neglected SRs"=w521:T13[])  [unwired: 6 in]
        n241 = control-ref of="Open SRs"() -> (w529:refnum<vi>)
        n242 = control-ref of="Neglected SRs"() -> (w528:refnum<vi>)
        n243 = control-ref of="SR Summary"() -> (w530:refnum<vi>)
        n244 = call "PopulateTree(SubVI).vi"("Tree Control reference"=w530, "Array"=w524, "Error In"=w523, "Filter By AE Name"=w511) -> ("Error Out"=w517:errorcluster)  [unwired: 6 in]
        n245 = call "PopulateTree(SubVI).vi"("Tree Control reference"=w529, "Array"=w525, "Error In"=w526) -> ("Error Out"=w520:errorcluster)  [unwired: 7 in]
        n246 = call "PopulateTree(SubVI).vi"("Tree Control reference"=w528, "Array"=w521, "Error In"=w522) -> ("Error Out"=w519:errorcluster)  [unwired: 7 in]
        n247 = Merge Errors(w517, w520, w519) -> (w518:errorcluster)
      }
      frame "SaveNeglectedToFile" {
      }
      frame "RemapAENames" {
        n248 = Unbundle By Name(w543) -> ("Report DVR"=w538:refnum<data-value>, "AE-NamesMapping"=w541:T12, "CISCO Agents"=w536:string[])
        n249 = call "FindUniqueAEs(SubVI).vi"("Report DVR"=w538) -> ("AE names array Out"=w537:string[])  [unwired: 10 in]
        n250 = call "RemapAENames.vi"("error in (no error)"=w542, "CISCO Agents"=w536, "Current AE-NamesMapping"=w541, "AE-NamesRaw (Repport)"=w537) -> ("error out"=w540:errorcluster)  [unwired: 7 in]
        n251 = call "ProcessQ_Send(SubVI).vi"("error in (no error)"=w540, "Command"=Command_Enum."LoadReport") -> ("error out"=w539:errorcluster)  [unwired: 9 in]
      }
      frame "DisplayAEStats" {
        n252 = Unbundle By Name(w562) -> ("Report DVR"=w551:refnum<data-value>, "Controls.Cluster Controls.Configuration"=w549:refnum<vi>)
        n253 = property class="Clust"(reference=w549, error in=w550) -> (error out=w545:errorcluster, "Value"=w548:variant)  [unwired: 1 out]
        n254 = Variant To Data(error in=w545, type=T6 {"AE"="", "Period"={"Start Date"=timestamp(0 s since 1904-01-01), "End Date"=timestamp(0 s since 1904-01-01)}} ("Configuration"), Variant=w548) -> (data=w546:T6, error out=w544:errorcluster)
        n255 = Unbundle By Name(w546) -> ("Period"=w559:T14, "AE"=w553:string)
        n256 = call "GetSRsbyStatus.vi"("Period"=w559, "Statuses"=string[] ["Resolved", "Presumed Resolved", "RMA Closed", "Forum Resolved AE", "Potentially Resolved", "RMA Approved for Return"], "Error In"=w544, "Report DVR in"=w551) -> ("Error Out"=w560:errorcluster, "SRs Out"=w554:T13[])  [unwired: 5 in, 1 out]
        n257 = call "GetAEStats.vi"("Error In"=w560, "SRs Out"=w554, "AE Name"=w553) -> ("Error Out"=w556:errorcluster, "Survey Data Out  (Table)"=→"AE Statistics":string[][])  [unwired: 5 in, 2 out]
        n258 = control-ref of="SR View"() -> (w557:refnum<vi>)
        n259 = call "PopulateTree(SubVI).vi"("Tree Control reference"=w557, "Array"=w554, "Display Neglected Status? (T)"=FALSE, "Error In"=w556, "Filter By AE Name"=w553) -> ("Error Out"=w555:errorcluster)  [unwired: 5 in]
      }
      frame "ScreenPop" {
        n260 = Variant To Data(error in=w568, type="", Variant=w567) -> (data=w564:string, error out=w565:errorcluster)
        n261 = call "ScreenPop(SubVI).vi"("Error In"=w565, "SR #"=w564) -> ("error out"=w563:errorcluster)  [unwired: 9 in]
      }
      frame "GetSRNotes" {
        n262 = Variant To Data(error in=w576, type="", Variant=w573) -> (data=w574:string, error out=w575:errorcluster)
        n263 = call "GetSRBody.vi"("Error In"=w575, "SR #"=w574) -> ("Error Out"=w578:errorcluster, "SR Notes"=→"SR Notes":string[], "Documents Used"=→"Documents Linked":string[][], "Documents Marked as Solution"=→"Documents marked as solution":string[][])  [unwired: 6 in]
      }
      frame "ClipboardCopy" {
        n264 = Variant To Data(error in=w585, type="", Variant=w580) -> (data=w581:string, error out=w583:errorcluster)
        n265 = invoke class="App" method="Clipboard.Write"(error in=w583, "Param 0"=w581) -> (error out=w582:errorcluster)  [unwired: 2 in, 3 out]
      }
      frame "UpdateCiscoAgentsView" {
        n266 = Unbundle By Name(w601) -> ("CISCO Agents"=w602:string[])
        n267 = Unbundle By Name(w601) -> ("Controls.Boolean.Update Required"=w600:refnum<vi>, "Controls.String Controls.New AEs"=w598:refnum<vi>, "Controls.Array Controls.Cisco Stats"=w597:refnum<vi>)
        n268 = Variant To Data(error in=w606, type=T2[] [] ("Cisco Stats"), Variant=w605) -> (data=w589:T2[], error out=w596:errorcluster)
        n269 = for {
          tunnel: [w607] -> w603 mode=indexing
          tunnel: [w609] -> w588 mode=indexing if=w612
          tunnel: w602 -> [w611]
          tunnel: w589 -> [w610] mode=indexing
          tunnel: [w609] -> w587 mode=indexing
          n270 = Unbundle By Name(w610) -> ("Agent Name"=w609:string)
          n271 = Search 1D Array(1D array=w611, element=w609) -> (index of element=w608:i32)  [unwired: 1 in]
          n272 = Greater Or Equal To 0?(x=w608) -> (x >= 0?=w607:bool)
          n273 = Not(x=w607) -> (.not. x?=w612:bool)
        }
        n274 = And Array Elements(Boolean array=w603) -> (logical AND=w591:bool)
        n275 = Not(x=w591) -> (.not. x?=w599:bool)
        n276 = property class="Bool (strict)"(reference=w600, error in=w596, "Value"=w599) -> (error out=w595:errorcluster)  [unwired: 1 out]
        n277 = property class="CmbBox"(reference=w598, error in=w596, "Strings[]"=w588) -> (error out=w594:errorcluster)  [unwired: 1 out]
        n278 = property class="Arr (strict)"(reference=w597, error in=w596, "Value"=w589) -> (error out=w593:errorcluster)  [unwired: 1 out]
        n279 = Bundle By Name(cluster=w601, "CISCO Agents"=w587) -> (w604:T7)
        n280 = Merge Errors(w595, w594, w593) -> (w592:errorcluster)
      }
      frame "UpdateKCSColorCode" {
        n281 = Variant To Data(error in=w620, type=cluster{string, u32} {"", 0} ("output cluster"), Variant=w619) -> (data=w617:cluster{string, u32}, error out=w614:errorcluster)
        n282 = Unbundle(w617) -> (w615:string, w616:u32)
        n283 = Unbundle By Name(w622) -> ("Controls.Tree Controls.SR View"=w621:refnum<vi>)
        n284 = case shown="3" w616 {
          tunnel: w621 -> [_ w627 w632 w637]
          tunnel: w615 -> [_ w626 w631 w636]
          tunnel: w614 -> [w623 w625 w630 w635]
          tunnel: [w623 w624 w629 w634] -> w613
          frame 0, Default {
          }
          frame 1 {
            n285 = call "ColourElementTree(SubVI).vi"("Error In"=w625, "Color"=u32 1244961, "SR Number"=w626, "TreeControl in"=w627) -> ("Error Out"=w624:errorcluster)  [unwired: 7 in]
          }
          frame 2 {
            n286 = call "ColourElementTree(SubVI).vi"("Error In"=w630, "Color"=u32 15400704, "SR Number"=w631, "TreeControl in"=w632) -> ("Error Out"=w629:errorcluster)  [unwired: 7 in]
          }
          frame 3 {
            n287 = call "ColourElementTree(SubVI).vi"("Error In"=w635, "Color"=u32 6618880, "SR Number"=w636, "TreeControl in"=w637) -> ("Error Out"=w634:errorcluster)  [unwired: 7 in]
          }
        }
      }
      frame "Shutdown" {
        n288 = Unbundle By Name(w642) -> ("Report DVR"=w641:refnum<data-value>)
        n289 = call "CloseSRDataReference(SubVI).vi"("error in (no error)"=w639, "Report DVR"=w641) -> ("error out"=w640:errorcluster)  [unwired: 9 in]
      }
    }
    n290 = case shown="Error" w236 {
      selector: w236 -> [w239 w241]
      tunnel: [w239 w243] -> w235
      tunnel: w230 -> [w238 w245]
      tunnel: [w238 w245] -> w229
      frame No Error {
      }
      frame Error {
        n291 = call <vilib>:"Clear Errors.vi"("error in (no error)"=w241) -> ("error out"=w244:errorcluster)  [unwired: 5 in, 1 out]
        n292 = call "ProcessQ_Send(SubVI).vi"("High Priority"=TRUE, "error in (no error)"=w244, "Data"=w241, "Command"=Command_Enum."Error") -> ("error out"=w243:errorcluster)  [unwired: 7 in]
      }
    }
  }
  n293 = Merge Errors(w9, w10, w4, w3) -> (w8:errorcluster)
  n294 = call "Comm_FGV(SubVI).vi"("Enum"=FGV_Enum."Close", "error in (no error)"=w8) -> ("error out"=w6:errorcluster)  [unwired: 8 in, 1 out]
  n295 = disable-structure shown="RUN_TIME_ENGINE==True" {
    disable-tunnel: w6 -> [_ _]
    frame condition #0 (active) {
    }
    frame condition #1 {
      n296 = Quit LabVIEW() -> ()  [unwired: 1 in]
    }
  }
